vi "User Console.vi"(8 "error in (no error)":errorcluster) -> (0 "error out":errorcluster)   [LabVIEW 2017]
uses:
  Communication/Reference Action.ctl
panel:
  in  "Emergency":bool
  in  "Close Door":bool
  in  "Open Door":bool
  in  "1st Floor":bool
  in  "2nd Floor":bool
  in  "3rd Floor":bool
  in  "4th Floor":bool
  in  "1st Floor Up":bool
  in  "2nd Floor Up":bool
  in  "3rd Floor Up":bool
  in  "2nd Floor Down":bool
  in  "3rd Floor Down":bool
  in  "4th Floor Down":bool
  # "Elevator Call"
  # "Floor Selection"
  # "UI1\nUI2"
  # "Door Buttons"
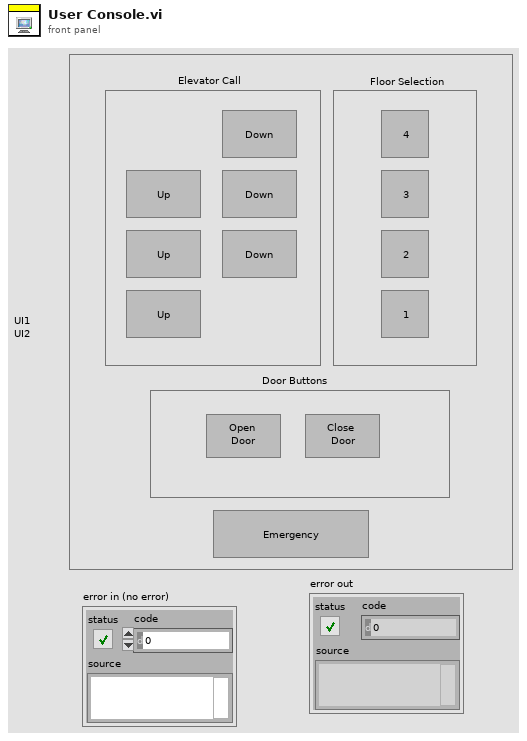
[diagram p1: front panel]
types:
  T1 = typedef "Reference Action.ctl" = enum16{"Set", "Get"}
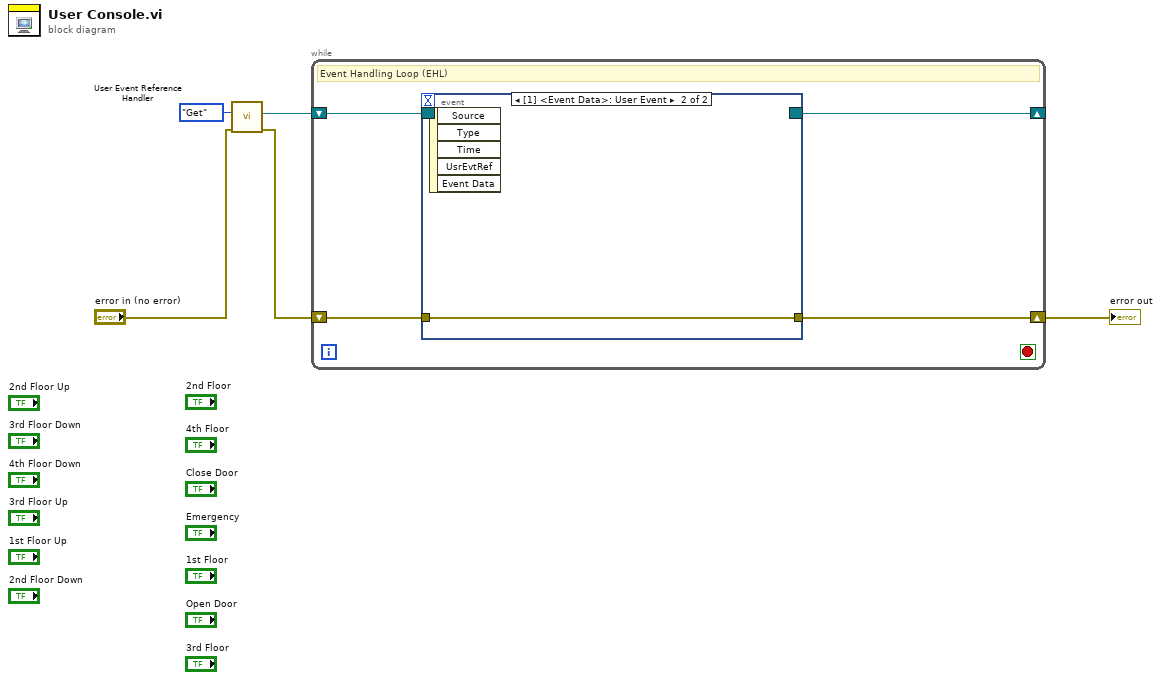
[diagram p0: block diagram]
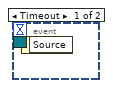
[diagram p2: hidden frame]
diagram:
  n1 = call "User Event Reference Handler.vi"("Reference Action"=Reference_Action."Get", "Error In"="error in (no error)") -> ("Error Out"=w2:errorcluster, "Event Registration Refnum Out"=w5:refnum<event-registration>)  [unwired: 7 in, 1 out]
  n2 = while {
    shift-right: [w9] -> _
    shift-left: w5 -> [w6]
    shift-right: [w7] -> w1
    shift-left: w2 -> [w8]
    stop <- _ stop-if-true
    # "Event Handling Loop (EHL)"
    n3 = event shown="[1] <Event Data>: User Event" {
      selector: w6 -> [_ _]
      dyn-events: [_ _] -> w9
      timeout: _ -> [_ _]
      tunnel: w8 -> [_ w10]
      tunnel: [_ w10] -> w7
      event Timeout {
        n4 = event-data() -> ()  [unwired: 1 in, 1 out]
      }
      event User Event {
        n5 = event-data() -> ()  [unwired: 1 in, 5 out]
      }
    }
  }
  "error out" <- w1
